vi "Close.vi"(11 "Channel Data In":T1) -> (3 "Channel Data":T1)   [LabVIEW 2022 SP3, in "Flex.lvlib"]
uses:
  Flex.lvlib
  Channel Data.ctl
  Element Info.ctl
  Element.ctl
  Event Data.ctl
  Writer Data.ctl
  Queue Data.ctl
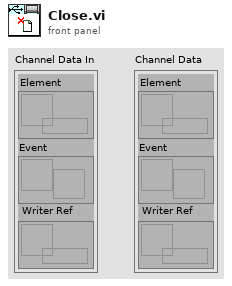
[diagram p1: front panel]
types:
  T1 = typedef "Flex.lvlib/Channel Data.ctl" = cluster{"Element":refnum<data-value>, "Event":refnum<user-event>, "Writer Ref":refnum<data-value>}
  T2 = typedef "Flex.lvlib/Event Data.ctl" = cluster{"Value":T3, "Closed":bool}
  T3 = typedef "Flex.lvlib/Element.ctl" = dbl
  T4 = typedef "Flex.lvlib/Writer Data.ctl" = cluster{"Lossless":refnum<queue>[], "Events":bool, "Lossy":bool}
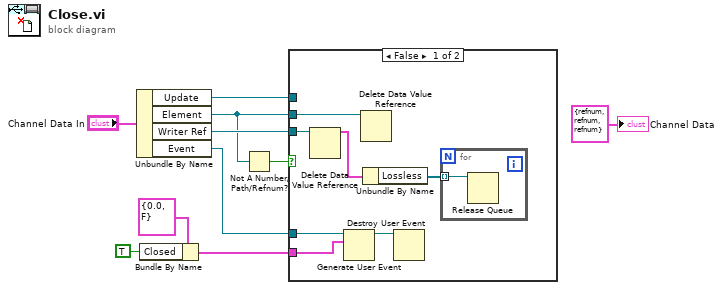
[diagram p0: block diagram]
diagram:
  n1 = Unbundle By Name("Channel Data In") -> ("Update"=w7:refnum<k4>, "Element"=w6:refnum<data-value>, "Writer Ref"=w8:refnum<data-value>, "Event"=w1:refnum<user-event>)
  n2 = Bundle By Name(cluster=T2 {"Value"=0.0, "Closed"=FALSE} ("Event Data"), "Closed"=TRUE) -> (w2:T2)
  n3 = Not A Number/Path/Refnum?(number/path/refnum=w6) -> (NaN/Path/Refnum?=w5:bool)
  n4 = case shown="False" w5 {
    tunnel: w8 -> [w17 _]
    tunnel: w7 -> [_ _]
    tunnel: w6 -> [w15 _]
    tunnel: w2 -> [w14 _]
    tunnel: w1 -> [w12 _]
    frame False {
      n5 = Delete Data Value Reference(data value reference=w17) -> (data value=w16:T4)  [unwired: 1 in, 1 out]
      n6 = Generate User Event(user event=w12, event data cluster=w14) -> (user event out=w13:refnum<user-event>)  [unwired: 2 in, 1 out]
      n7 = Delete Data Value Reference(data value reference=w15) -> ()  [unwired: 1 in, 2 out]
      n8 = Unbundle By Name(w16) -> ("Lossless"=w11:refnum<queue>[])
      n9 = Destroy User Event(user event=w13) -> ()  [unwired: 1 in, 1 out]
      n10 = for {
        tunnel: w11 -> [w18] mode=indexing
        n11 = Release Queue(queue=w18) -> ()  [unwired: 2 in, 3 out]
      }
    }
    frame True {
      # "Already closed"
    }
  }
  "Channel Data" <- T1 {"Element"=refnum, "Event"=refnum, "Writer Ref"=refnum} ("Channel Data")
